vi "getDeviceHandle.vi"(8 "error in (no error)":errorcluster, 11 "Model in":refnum<class "Model.lvclass">) -> (0 "error out":errorcluster, 2 "Device":i32, 3 "Model out":refnum<class "Model.lvclass">)   [LabVIEW 2016, in "Model.lvclass"]
uses:
  Model.lvclass
  Model.lvclass/Model.ctl
  ss_sedspectrometer/SEDSpectrometer/FiberSpectrograph.lvclass
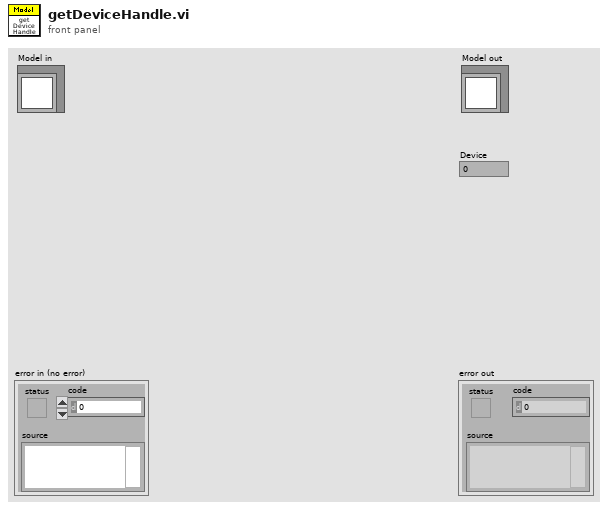
[diagram p1: front panel]
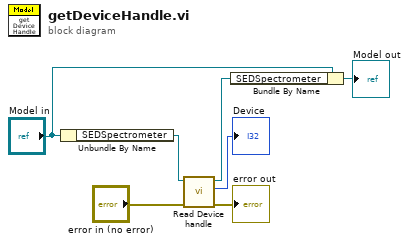
[diagram p0: block diagram]
diagram:
  n1 = Unbundle By Name("Model in") -> ("SEDSpectrometer"=w7:refnum<class "FiberSpectrograph.lvclass">)
  n2 = call-dynamic "Read Device handle.vi"("error in (no error)"="error in (no error)", "SEDSpectrometer in"=w7) -> ("error out"=→"error out":errorcluster, "Device handle"=→"Device":i32, "SEDSpectrometer out"=w4:refnum<class "FiberSpectrograph.lvclass">)  [unwired: 7 in]
  n3 = Bundle By Name(cluster="Model in", "SEDSpectrometer"=w4) -> (→"Model out":refnum<class "Model.lvclass">)
